vi "JSON to LVObject - Error in Serializable Class - Returns Same Error.vi"() -> ()   [LabVIEW 2017, in "JSON Serializable Serializer Tests.lvlib"]
uses:
  JSON Serializable Serializer Tests.lvlib
  JSON Serializable Serializer/JSON Serializable Serializer.lvclass
  <vilib>/Utility/error.llb/Error Cluster From Error Code.vi
  <vilib>/addons/_JKI Toolkits/Caraya/classes/Assert/Assert Equal Value_Variant.vi
  <vilib>/ErrorRing/Error Ring.xnode
  <vilib>/addons/_JKI Toolkits/Caraya/classes/Test/Test.lvclass
  <vilib>/addons/_JKI Toolkits/Caraya/classes/Assert/Assert.lvclass
  Mock JSON Serializable/Mock JSON Serializable.lvclass
panel:
  out "error out":errorcluster
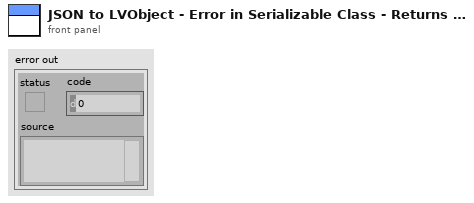
[diagram p1: front panel]
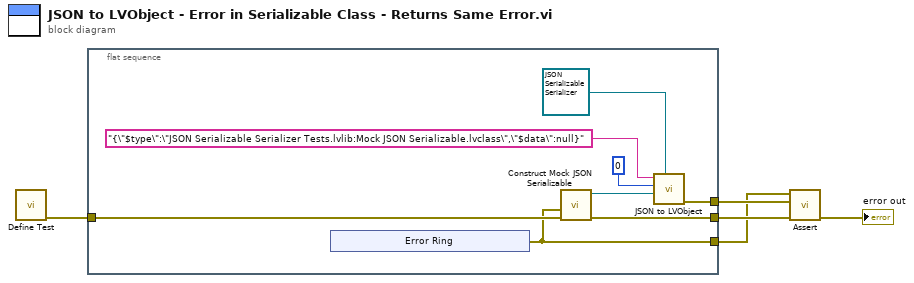
[diagram p0: block diagram]
diagram:
  n1 = call <vilib>:"Define Test.vi"() -> ("error out"=w5:errorcluster)  [unwired: 11 in]
  n2 = flat-sequence {
    tunnel: [w8] -> w3
    tunnel: w5 -> [w10]
    tunnel: [w7] -> w2
    tunnel: [w6] -> w1
    frame #0 {
      n3 = xnode "Error Ring"() -> ("error out"=w6:errorcluster)
      n4 = call "Construct Mock JSON Serializable.vi"("error in (no error)"=w10, "From/To JSON <error out> (no error)"=w6) -> ("error out"=w8:errorcluster, "Mock JSON Serializable"=w9:refnum<class "Mock JSON Serializable.lvclass">)  [unwired: 8 in]
      n5 = call-dynamic "JSON to LVObject.vi"("JSON Serializable Serializer in"=refnum<class "JSON Serializable Serializer.lvclass"> refnum ("JSON Serializer.lvclass"), "Object Type"=w9, "Offset"=0, "JSON"="{\"$type\":\"JSON Serializable Serializer Tests.lvlib:Mock JSON Serializable.lvclass\",\"$data\":null}") -> ("error out"=w7:errorcluster)  [unwired: 6 in, 1 out]
    }
  }
  n6 = call-poly <vilib>:"Assert.vi"("error in (no error)"=w3, "Y"=w2, "X"=w1) -> ("error out"=→"error out":errorcluster)  [unwired: 8 in]
